vi "Get number of primes in a thousand.vi"(8 "error in (no error)":errorcluster, 10 "Bin size":i32=1000, 11 "List of primes (sorted ascending)":i32[](array[numeric])=array[78498 elements]) -> (0 "error out":errorcluster, 1 "Waveform Graph":i32[](graph), 2 "Number of bins":i32, 3 "Primes per bin":i32[](array[numeric]))   [LabVIEW 2021, in "Numeric Utilities.lvlib"]
uses:
  Numeric Utilities.lvlib
  <userlib>/_OpenG.lib/array/array.llb/Delete Elements from 1D Array (I32)__ogtk.vi
  Named Timers/Named Timers.lvlib
panel:
  out "Elapsed time (s)":dbl
  out "Remaining elements":i32
  in  "Loop period (ms)":u32
  in  "Stop Button":bool
  out "2D array":i32[][](array[numeric])
  out "Lower limit":i32
  out "Upper limit":i32
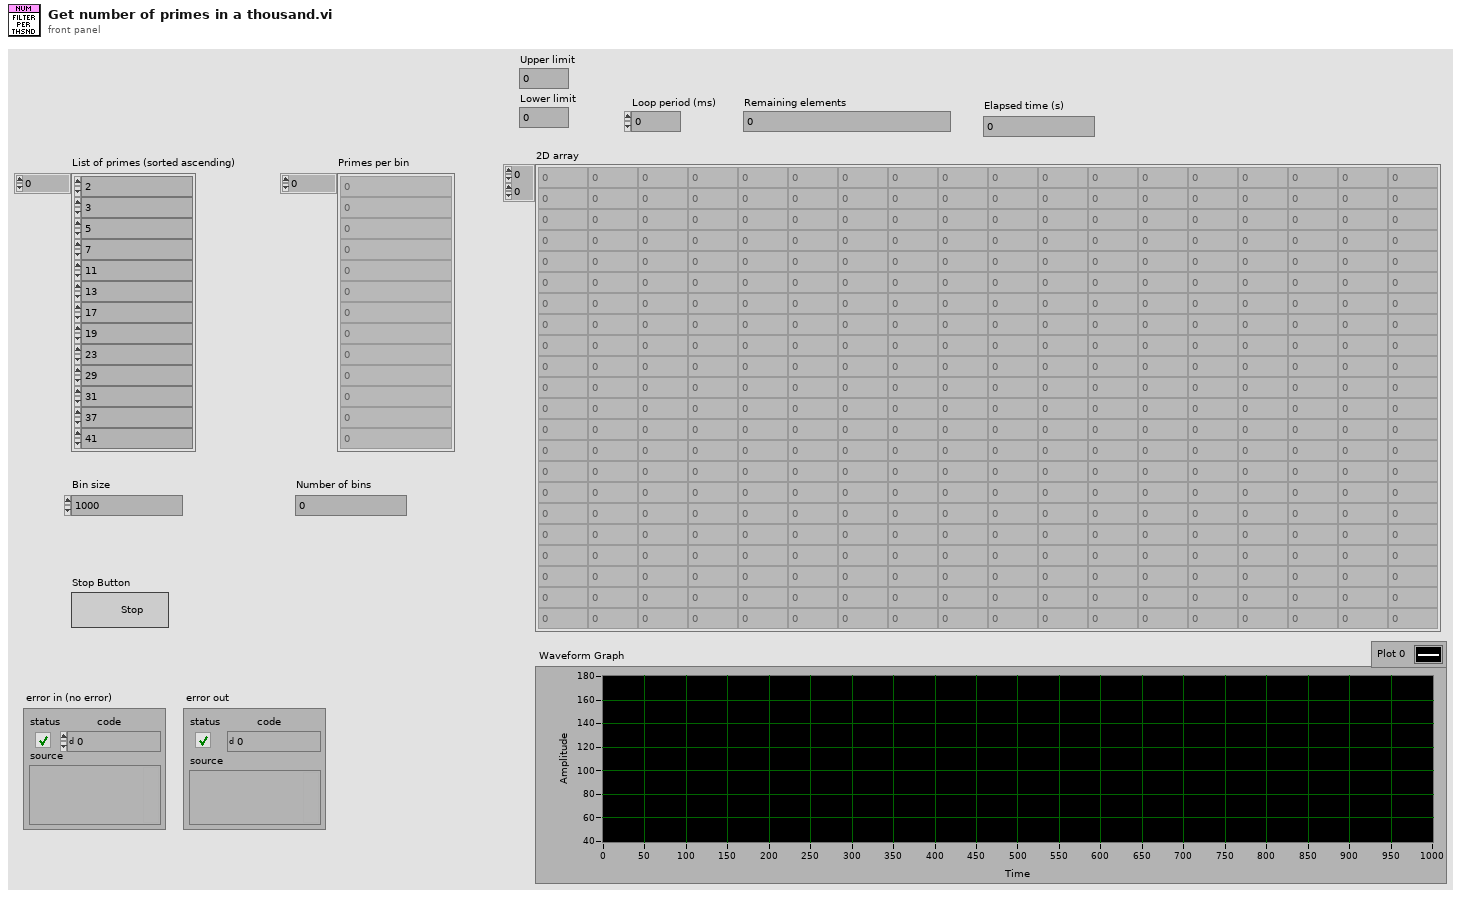
[diagram p1: front panel]
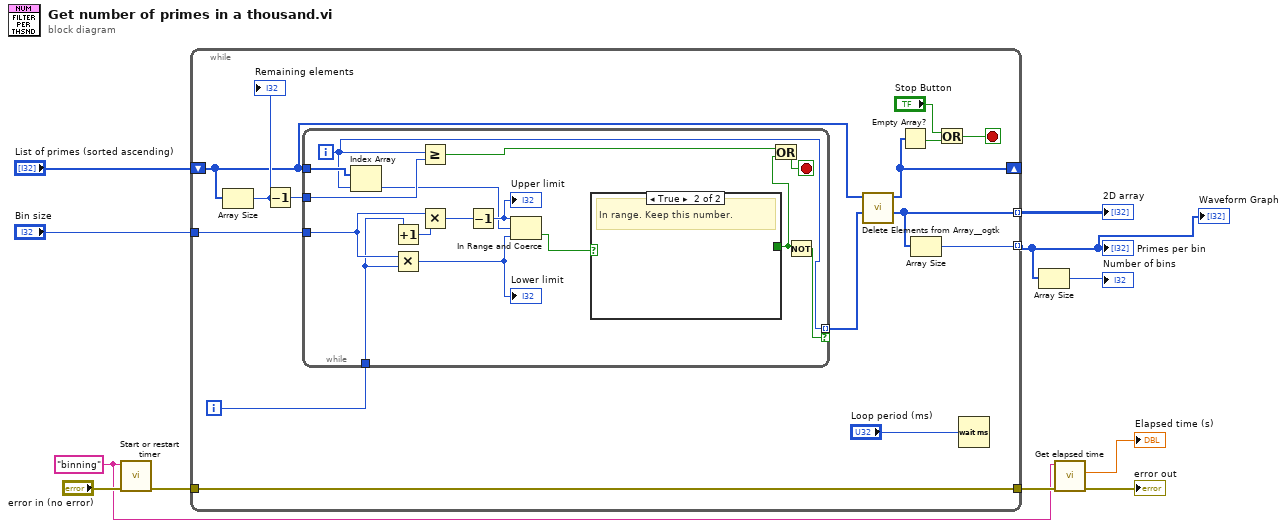
[diagram p0: block diagram]
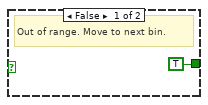
[diagram p2: hidden frame]
diagram:
  w2 = "binning" ("Timer name")
  n1 = call "Start or restart timer.vi"("error in (no error)"="error in (no error)", "Timer name"=w2) -> ("error out"=w4:errorcluster)  [unwired: 9 in]
  n2 = while {
    shift-right: [w17] -> _
    shift-left: "List of primes (sorted ascending)" -> [w21]
    tunnel: "Bin size" -> [w25]
    tunnel: [w19] -> w9 mode=indexing
    tunnel: [w18] -> w7 mode=indexing
    tunnel: w4 -> [w12]
    tunnel: [w12] -> w5
    i -> [w24]
    stop <- w14 stop-if-true
    n3 = Array Size(array=w21) -> (size(s)=w23:i32)
    "Remaining elements" <- w23
    n4 = Decrement(x=w23) -> (x-1=w22:i32)
    n5 = while {
      tunnel: w25 -> [w40]
      tunnel: w24 -> [w39]
      tunnel: w21 -> [w28]
      tunnel: w22 -> [w33]
      tunnel: [w27] -> w20 mode=indexing if=w29
      i -> [w27]
      stop <- w31 stop-if-true
      n6 = Index Array(array=w28, index=w27) -> (element=w26:i32)
      n7 = Increment(x=w39) -> (x+1=w38:i32)
      n8 = Multiply(x=w40, y=w39) -> (x*y=w35:i32)
      "Lower limit" <- w35
      n9 = Greater Or Equal?(x=w27, y=w33) -> (x >= y?=w32:bool)
      n10 = Multiply(x=w40, y=w38) -> (x*y=w37:i32)
      n11 = Decrement(x=w37) -> (x-1=w36:i32)
      "Upper limit" <- w36
      n12 = In Range and Coerce(upper limit=w36, x=w26, lower limit=w35) -> (In Range?=w34:bool)  [unwired: 1 out]
      n13 = case shown="True" w34 {
        tunnel: [TRUE _] -> w30
        frame False {
          # "Out of range. Move to next bin."
        }
        frame True {
          # "In range. Keep this number."
        }
      }
      n14 = Or(x=w32, y=w30) -> (x .or. y?=w31:bool)
      n15 = Not(x=w30) -> (.not. x?=w29:bool)
    }
    n16 = call-poly <userlib>:"Delete Elements from Array__ogtk.vi"("indices"=w20, "array"=w21) -> ("deleted elements"=w19:i32[], "array w/ subset deleted"=w17:i32[])  [unwired: 8 in]
    n17 = Empty Array?(array=w17) -> (empty?=w16:bool)
    n18 = Array Size(array=w19) -> (size(s)=w18:i32)
    n19 = Or(x="Stop Button", y=w16) -> (x .or. y?=w14:bool)
    n20 = Wait (ms)(milliseconds to wait="Loop period (ms)") -> ()  [unwired: 1 out]
  }
  "Primes per bin" <- w7
  "2D array" <- w9
  "Waveform Graph" <- w7
  n21 = Array Size(array=w7) -> (size(s)=→"Number of bins":i32)
  n22 = call "Get elapsed time.vi"("error in (no error)"=w5, "Timer name"=w2) -> ("error out"=→"error out":errorcluster, "Elapsed time (s)"=→"Elapsed time (s)":dbl)  [unwired: 6 in, 2 out]
